vi "ProcessStartupMetrics.vi"(8 "error in (no error)":errorcluster, 9 "Startup Analysis Configuration":T4, 11 "data in":T1) -> (0 "error out":errorcluster)   [LabVIEW 2017, in "McsaStartupAnalysis.lvlib"]
uses:
  <vilib>/addons/InsightCM/Devices/Shared/Mcsa/McsaStartupAnalysis/McsaStartupAnalysis.lvlib
  <vilib>/addons/InsightCM/Devices/Shared/Mcsa/McsaStartupAnalysis/controls/Config.ctl
  <vilib>/addons/InsightCM/Devices/Shared/Mcsa/McsaStartupAnalysis/controls/Group.ctl
  <vilib>/addons/InsightCM/Devices/Shared/Mcsa/McsaStartupAnalysis/controls/ChannelForStartup.ctl
  <vilib>/addons/InsightCM/Devices/Shared/Mcsa/McsaStartupAnalysis/controls/StartupFeature.ctl
  <vilib>/addons/InsightCM/Devices/Shared/Mcsa/McsaStartupAnalysis/controls/MotorInfo.ctl
  <vilib>/addons/InsightCM/Devices/Shared/Common/FileFlow/controls/data_eventRef.ctl
  <vilib>/addons/InsightCM/Devices/Shared/Common/DataEvent/controls/EventReference.ctl
  <vilib>/addons/InsightCM/Devices/Shared/Common/DataEvent/controls/Event.ctl
  <vilib>/addons/InsightCM/MessageBus/Base/controls/DataEvent.ctl
  <vilib>/addons/InsightCM/MessageBus/Base/controls/KeyValuePair.ctl
  <vilib>/addons/InsightCM/Devices/Shared/Common/DataEvent/controls/DataSet.ctl
  <vilib>/addons/InsightCM/MessageBus/Base/controls/DataSetMetadata.ctl
  <vilib>/addons/InsightCM/MessageBus/Base/controls/TrendPoint.ctl
  <vilib>/addons/InsightCM/MessageBus/Base/controls/TrendAlarmUpdate.ctl
  <vilib>/addons/InsightCM/MessageBus/Base/controls/TrendAlarmTransition.ctl
  <vilib>/addons/PointValueMap/controls/PointMap.ctl
  <vilib>/addons/InsightCM/Utilities/PropertyHelpers/PropertyHelpers.lvlib
  <vilib>/addons/InsightCM/Devices/Shared/Common/DataEvent/DataEvent.lvlib
  <vilib>/addons/PointValueMap/PointValueMap.lvlib
  <vilib>/addons/InsightCM/Devices/Shared/Common/FileFlow/FileFlow.lvlib
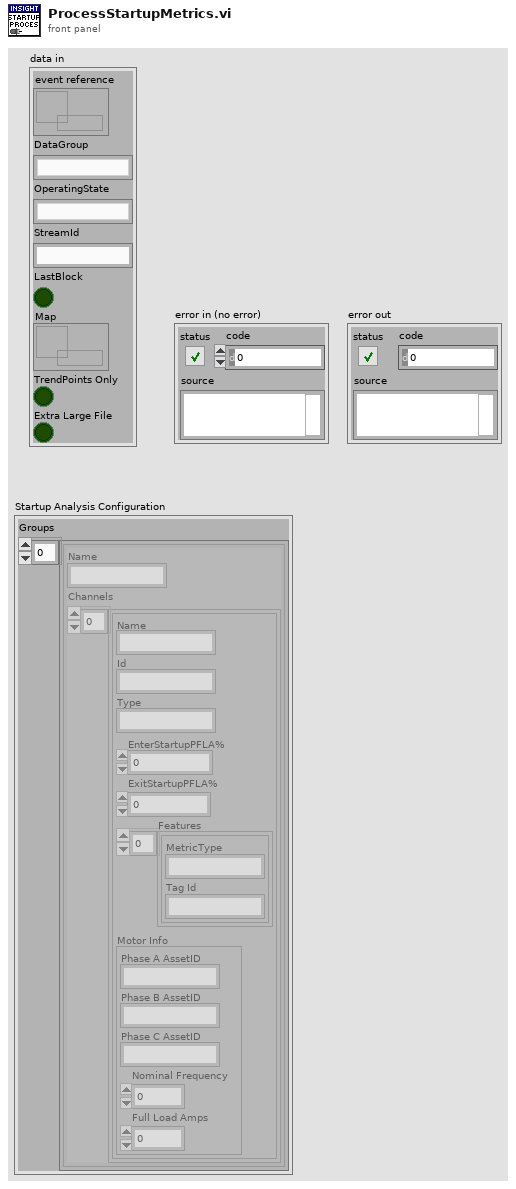
[diagram p1: front panel]
types:
  T1 = typedef "FileFlow.lvlib/data_eventRef.ctl" = cluster{"event reference":T2, "DataGroup":string, "OperatingState":string, "StreamId":string, "LastBlock":bool, "Map":T3, "TrendPoints Only":bool, "Extra Large File":bool}
  T2 = typedef "DataEvent.lvlib/EventReference.ctl" = refnum<data-value>
  T3 = typedef "PointValueMap.lvlib/PointMap.ctl" = refnum<data-value>
  T4 = typedef "McsaStartupAnalysis.lvlib/Config.ctl" = cluster{"Groups":T5[]}
  T5 = typedef "McsaStartupAnalysis.lvlib/Group.ctl" = cluster{"Name":string, "Channels":T6[]}
  T6 = typedef "McsaStartupAnalysis.lvlib/ChannelForStartup.ctl" = cluster{"Name":string, "Id":string, "Type":string, "EnterStartupPFLA%":dbl, "ExitStartupPFLA%":dbl, "Features":T7[], "Motor Info":T8}
  T7 = typedef "McsaStartupAnalysis.lvlib/StartupFeature.ctl" = cluster{"MetricType":string, "Tag Id":string}
  T8 = typedef "McsaStartupAnalysis.lvlib/MotorInfo.ctl" = cluster{"Phase A AssetID":string, "Phase B AssetID":string, "Phase C AssetID":string, "Nominal Frequency":dbl, "Full Load Amps":dbl}
  T9 = typedef "DataEvent.lvlib/Event.ctl" = cluster{"DataEvent":T10, "DataSets":T12[], "TrendPoints":T14[], "Alarms":T15[]}
  T10 = typedef "DataEvent.ctl" = cluster{"Id":string, "AssetNodeId":string, "Timestamp":i64, "Props":T11[]}
  T11 = typedef "KeyValuePair.ctl" = cluster{"Key":string, "Value":string}
  T12 = typedef "DataEvent.lvlib/DataSet.ctl" = cluster{"DataSetMetadata":T13, "Values":sgl[], "Values DVR":refnum<data-value>}
  T13 = typedef "DataSetMetadata.ctl" = cluster{"Id":string, "DataEventId":string, "AssetNodeId":string, "Type":string, "T0":i64, "Props":T11[]}
  T14 = typedef "TrendPoint.ctl" = cluster{"TrendPointId":string, "DataEventId":string, "Timestamp":i64, "Value":dbl, "Props":T11[]}
  T15 = typedef "TrendAlarmUpdate.ctl" = cluster{"RuleId":string, "Transition":T16}
  T16 = typedef "TrendAlarmTransition.ctl" = cluster{"At":i64, "Severity":i32, "Value":dbl}
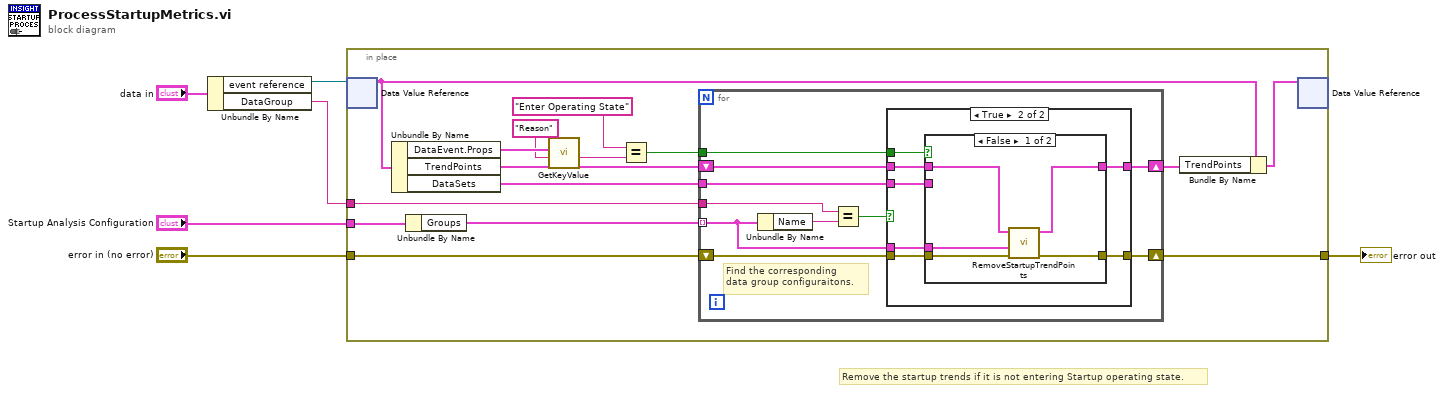
[diagram p0: block diagram]
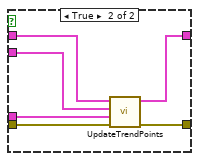
[diagram p3: hidden frame]
diagram:
  # "Remove the startup trends if it is not entering Startup operating state."
  n1 = Unbundle By Name("data in") -> ("event reference"=w4:T2, "DataGroup"=w3:string)
  n2 = in-place {
    in-place-border: "Startup Analysis Configuration" -> [w20]
    in-place-border: w3 -> [w15]
    in-place-border: "error in (no error)" -> [w13]
    in-place-border: [w12] -> w1
    n3 = in-place-dvr #1(w4) -> (w18:T9)  [unwired: 1 out]
    n4 = Unbundle By Name(w18) -> ("DataEvent.Props"=w10:T11[], "TrendPoints"=w17:T14[], "DataSets"=w14:T12[])
    n5 = Unbundle By Name(w20) -> ("Groups"=w21:T5[])
    n6 = call <vilib>:"GetKeyValue.vi"("key"="Reason" ("x"), "key value pairs"=w10) -> ("value"=w8:string)  [unwired: 7 in, 2 out]
    n7 = Equal?(x="Enter Operating State", y=w8) -> (x = y?=w7:bool)
    n8 = for {
      tunnel: w21 -> [w30] mode=indexing
      shift-right: [w28] -> w16
      shift-left: w17 -> [w29]
      tunnel: w15 -> [w27]
      tunnel: w14 -> [w26]
      shift-right: [w24] -> w12
      shift-left: w13 -> [w25]
      tunnel: w7 -> [w22]
      # "Find the corresponding\ndata group configuraitons."
      n9 = Unbundle By Name(w30) -> ("Name"=w31:string)
      n10 = Equal?(x=w27, y=w31) -> (x = y?=w23:bool)
      n11 = case shown="True" w23 {
        tunnel: w30 -> [_ w40]
        tunnel: w29 -> [w33 w39]
        tunnel: [w33 w38] -> w28
        tunnel: w26 -> [_ w37]
        tunnel: w25 -> [w32 w36]
        tunnel: [w32 w35] -> w24
        tunnel: w22 -> [_ w34]
        frame False {
        }
        frame True {
          n12 = case shown="False" w34 {
            tunnel: w40 -> [w44 w51]
            tunnel: w39 -> [w42 w50]
            tunnel: [w41 w49] -> w38
            tunnel: w37 -> [_ w48]
            tunnel: w36 -> [w45 w47]
            tunnel: [w43 w46] -> w35
            frame False {
              n13 = call <vilib>:"RemoveStartupTrendPoints.vi"("error in (no error)"=w45, "Group"=w44, "TrendPoints in"=w42) -> ("error out"=w43:errorcluster, "TrendPoints out"=w41:T14[])  [unwired: 7 in]
            }
            frame True {
              n14 = call <vilib>:"UpdateTrendPoints.vi"("error in (no error)"=w47, "Group"=w51, "DataSets"=w48, "TrendPoints in"=w50) -> ("error out"=w46:errorcluster, "TrendPoints out"=w49:T14[])  [unwired: 6 in]
            }
          }
        }
      }
    }
    n15 = Bundle By Name(cluster=w18, "TrendPoints"=w16) -> (w19:T9)
    n16 = in-place-dvr #1(w19) -> ()  [unwired: 2 out]
  }
  "error out" <- w1
